vi "is executable.vi"() -> (0 "Is Executable?":bool)   [LabVIEW 2020, in "Reusable Library.lvlib"]
doc: "This VI will check if the application on development environment or run time environment. Returns true if EXE (Run time environment)"
uses:
  Reusable Library.lvlib
panel:
  # "Samuel J\n     Measurement Engineer\n     Certified LabVIEW Architect\n     Vestas Technology R&D Chennai"
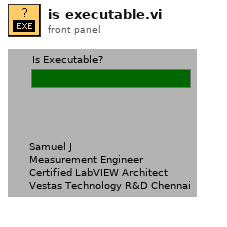
[diagram p1: front panel]
types:
  T1 = enum32{"invalid app kind", "Development System", "Run Time System", "Student Edition", "Embedded LabVIEW", "Evaluation", "Custom"}
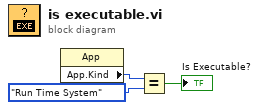
[diagram p0: block diagram]
diagram:
  n1 = property class="App"() -> ("App.Kind"=w3:T1)  [unwired: 2 in, 2 out]
  n2 = Equal?(x=w3, y=T1."Run Time System" ("Application:Kind")) -> (x = y?=→"Is Executable?":bool)
